vi "IMAQ-GetMichelsonContrast.vi"(1 "Luma 2D Array":dbl[][](array[numeric])) -> (0 "Michelson Contraste":dbl)   [LabVIEW 2010]
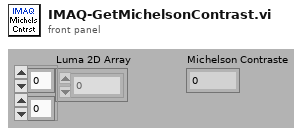
[diagram p1: front panel]
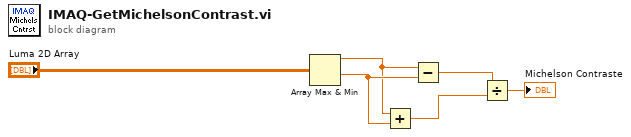
[diagram p0: block diagram]
diagram:
  n1 = Array Max & Min(array="Luma 2D Array") -> (max value=w2:dbl, min value=w3:dbl)  [unwired: 2 out]
  n2 = Add(x=w2, y=w3) -> (x+y=w4:dbl)
  n3 = Subtract(x=w2, y=w3) -> (x-y=w1:dbl)
  n4 = Divide(x=w1, y=w4) -> (x/y=→"Michelson Contraste":dbl)
